vi "WS1050_Extract Data From Scope_Filtered Signal.vi"(0 "file path":path=path "S:/_Employee_Folders/Andy temp/SN01/444AB_04__SN01_C1_S1_UP_Switch_Time_data.csv", 1 "60% Amp":dbl=0.6, 2 "95% Amp":dbl=0.95, 9 "Set Point for AMP":i32=7000, 11 "error in (no error)":errorcluster, 12 "90% Amp":dbl=0.9) -> (3 "AMP(v)":dbl=1.1, 4 "Amp(mv)":string, 6 "T2(us)":string, 8 "T3(us)":string, 10 "T1(us)":string, 15 "error out":errorcluster)   [LabVIEW 2012]
uses:
  <vilib>/Utility/file.llb/Read From Spreadsheet File (string).vi
  <vilib>/Analysis/2dsp.llb/Real FFT.vi
  <vilib>/Analysis/NI_AALPro.lvlib
panel:
  in  "Tab Control":enum32{"Control", "ST", "FFT"}(tab)
  in  "Enter Time(s)":dbl=0.0001
  in  "Full/Half":i32=2
  out "Signal":cluster{dbl, dbl}[](graph)
  out "Filtered Signal":cluster{dbl, dbl}[](graph)
  out "CLK":cluster{dbl, dbl}[](graph)
  out "Signal FFT":cluster{dbl, dbl}[](graph)
  out "Filtered Signal FFT":cluster{dbl, dbl}[](graph)
  # "Total Time is 10E-4"
  # "Note\nSample time is 10E-8\nTotal time is 10E-4"
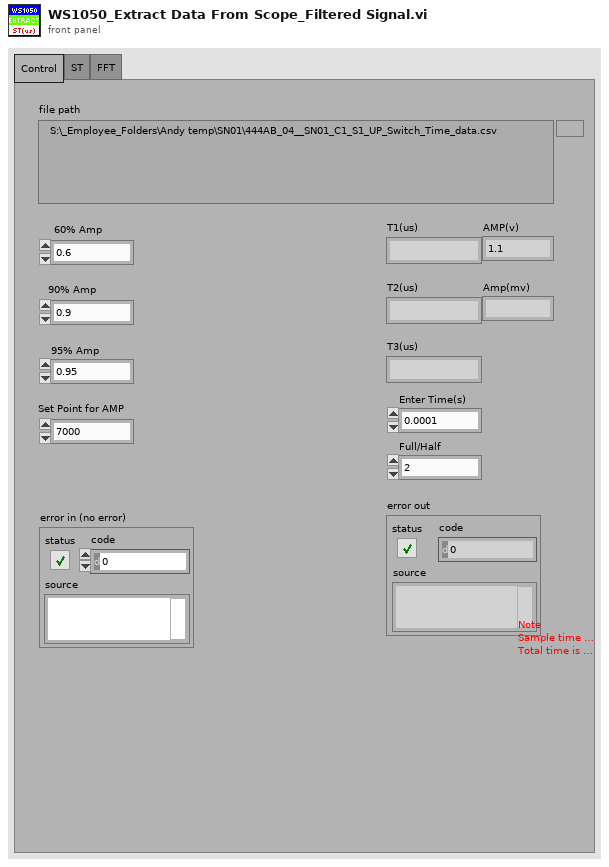
[diagram p1: front panel]
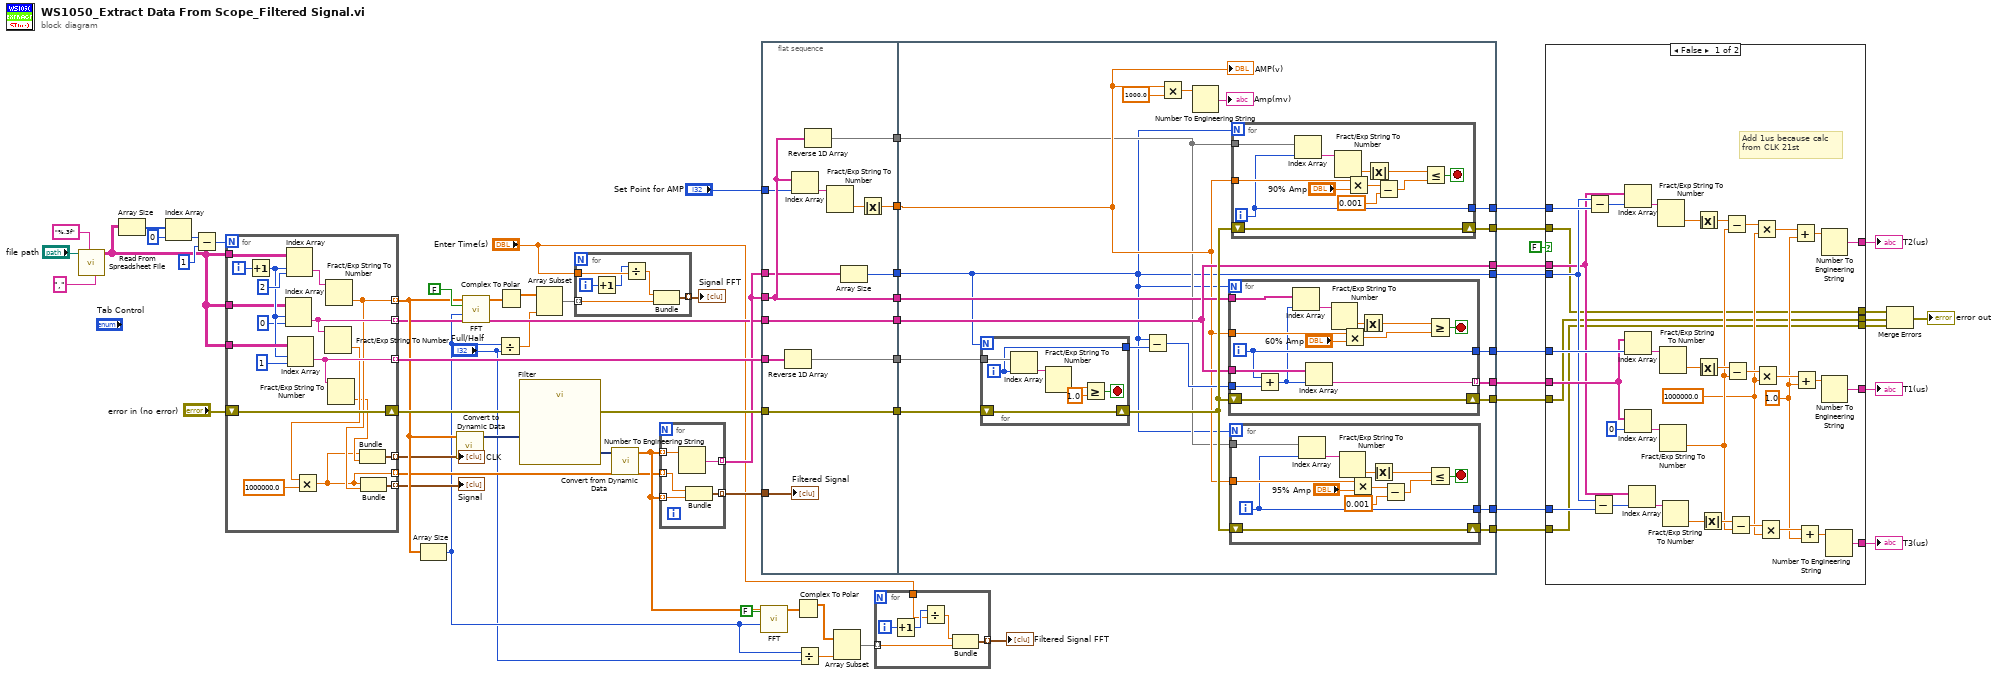
[diagram p0: block diagram]
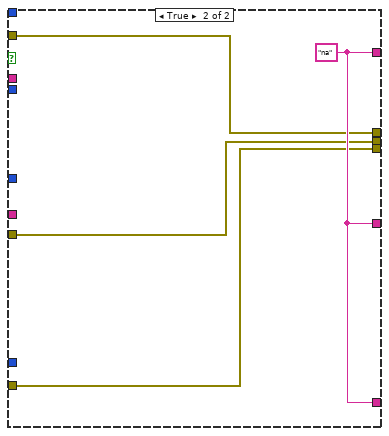
[diagram p2: hidden frame]
diagram:
  n1 = call-poly <vilib>:"Read From Spreadsheet File.vi"("delimiter (\\t)"="," ("delimiter (\\t)"), "format (%s)"="%.3f" ("format (%.3f)"), "file path (dialog if empty)"="file path") -> ("all rows"=w47:string[][])  [unwired: 4 in, 4 out]
  n2 = Array Size(array=w47) -> (size(s)=w60:i32[])
  n3 = Index Array(array=w60, index=0) -> (element=w58:i32)
  n4 = Subtract(x=w58, y=1) -> (x-y=w21:i32)
  n5 = for {
    N: w21 -> [_]
    tunnel: w47 -> [w82]
    tunnel: w47 -> [w79]
    tunnel: [w72] -> w55 mode=indexing
    tunnel: w47 -> [w76]
    tunnel: [w71] -> w18 mode=indexing
    shift-right: [w74] -> w30
    shift-left: "error in (no error)" -> [w74]
    tunnel: [w67] -> w19 mode=indexing
    tunnel: [w69] -> w16 mode=indexing
    tunnel: [w65] -> w14 mode=indexing
    tunnel: [w64] -> w12 mode=indexing
    i -> [w80]
    n6 = Increment(x=w80) -> (x+1=w77:i32)
    n7 = Index Array(array=w76, index (row)=w77, index (col)=0 ("disabled index (col)")) -> (element=w71:string)
    n8 = Index Array(array=w82, index (row)=w77, index (col)=2 ("disabled index (col)")) -> (element=w73:string)
    n9 = Index Array(array=w79, index (row)=w77, index (col)=1 ("disabled index (col)")) -> (element=w72:string)
    n10 = Fract/Exp String To Number(string=w71) -> (number=w68:dbl)  [unwired: 3 in, 1 out]
    n11 = Multiply(x=w68, y=1000000.0) -> (x*y=w65:dbl)
    n12 = Fract/Exp String To Number(string=w73) -> (number=w67:dbl)  [unwired: 3 in, 1 out]
    n13 = Fract/Exp String To Number(string=w72) -> (number=w66:dbl)  [unwired: 3 in, 1 out]
    n14 = Bundle(w65, w66) -> (w64:cluster{dbl, dbl})  [unwired: 1 in]
    n15 = Bundle(w65, w67) -> (w69:cluster{dbl, dbl})  [unwired: 1 in]
  }
  "Signal" <- w16
  "CLK" <- w12
  n16 = Array Size(array=w19) -> (size(s)=w4:i32)
  n17 = call "Convert to Dynamic Data"("Array"=w19) -> ("Dynamic Data Type"=w29:dynamicdata)  [unwired: 3 in]
  n18 = call-poly <vilib>:"FFT.vi"("FFT size"=w4, "shift?"=FALSE, "X"=w19) -> ("FFT {X}"=w24:cdb[])  [unwired: 7 in, 1 out]
  n19 = Divide(x=w4, y="Full/Half") -> (x/y=w3:dbl)
  n20 = Complex To Polar(r * e^(i*theta)=w24) -> (r=w6:dbl[])  [unwired: 1 out]
  n21 = call "Filter"("error in (no error)"=w30, "Signal"=w29) -> ("error out"=w28:errorcluster, "Filtered Signal"=w27:dynamicdata)  [unwired: 8 in]
  n22 = Array Subset(array=w6, length=w3) -> (w5:dbl[])  [unwired: 1 in]
  n23 = for {
    tunnel: w5 -> [w88] mode=indexing
    tunnel: [w87] -> w11 mode=indexing
    tunnel: "Enter Time(s)" -> [w84]
    i -> [w86]
    n24 = Increment(x=w86) -> (x+1=w83:i32)
    n25 = Divide(x=w83, y=w84) -> (x/y=w85:dbl)
    n26 = Bundle(w85, w88) -> (w87:cluster{dbl, dbl})  [unwired: 1 in]
  }
  "Signal FFT" <- w11
  n27 = call "Convert from Dynamic Data"("Dynamic Data Type"=w27) -> ("Array"=w15:dbl[])  [unwired: 3 in]
  n28 = for {
    tunnel: w15 -> [w93] mode=indexing
    tunnel: [w92] -> w26 mode=indexing
    tunnel: w15 -> [w91] mode=indexing
    tunnel: w14 -> [w90] mode=indexing
    tunnel: [w89] -> w13 mode=indexing
    n29 = Number To Engineering String(4:w93) -> (0:w92:string)  [unwired: 3 in]
    n30 = Bundle(w90, w91) -> (w89:cluster{dbl, dbl})  [unwired: 1 in]
  }
  n31 = call-poly <vilib>:"FFT.vi"("FFT size"=w4, "shift?"=FALSE, "X"=w15) -> ("FFT {X}"=w20:cdb[])  [unwired: 7 in, 1 out]
  n32 = flat-sequence {
    tunnel: w18 -> [w105]
    tunnel: w28 -> [w106]
    tunnel: w55 -> [w101]
    tunnel: [w106] -> w37
    tunnel: [w105] -> w36
    tunnel: w26 -> [w98]
    tunnel: [w102] -> w35
    tunnel: [w100] -> w34
    tunnel: [w99] -> w33
    tunnel: [w98] -> w32
    tunnel: [w97] -> w31
    tunnel: w26 -> [w96]
    tunnel: "Set Point for AMP" -> [w95]
    tunnel: w13 -> [w94]
    tunnel: [w126] -> w56
    tunnel: [w124] -> w52
    tunnel: [w123] -> w51
    tunnel: [w119] -> w49
    tunnel: [w118] -> w48
    tunnel: [w107] -> w43
    tunnel: [w113] -> w42
    tunnel: [w115] -> w46
    tunnel: [w114] -> w44
    tunnel: w37 -> [w125]
    tunnel: w36 -> [w113]
    tunnel: w35 -> [w110]
    tunnel: w34 -> [w109]
    tunnel: w33 -> [w108]
    tunnel: w32 -> [w111]
    tunnel: w31 -> [w107]
    frame #0 {
      n33 = Reverse 1D Array(array=w101) -> (reversed array=w100:string[])
      n34 = Index Array(array=w98, index=w95) -> (element=w103:string)
      n35 = Reverse 1D Array(array=w98) -> (reversed array=w99:string[])
      n36 = Fract/Exp String To Number(string=w103) -> (number=w104:dbl)  [unwired: 3 in, 1 out]
      n37 = Array Size(array=w96) -> (size(s)=w97:i32)
      n38 = Absolute Value(x=w104) -> (abs(x)=w102:dbl)
      "Filtered Signal" <- w94
    }
    frame #1 {
      n39 = for {
        N: w107 -> [_]
        tunnel: w109 -> [w171]
        tunnel: [w168] -> w117
        shift-right: [w166] -> w116
        shift-left: w125 -> [w166]
        i -> [w168]
        stop <- w169 stop-if-true
        n40 = Index Array(array=w171, index=w168) -> (element=w165:string)
        n41 = Fract/Exp String To Number(string=w165) -> (number=w167:dbl)  [unwired: 3 in, 1 out]
        n42 = Greater Or Equal?(x=w167, y=1.0) -> (x >= y?=w169:bool)
      }
      n43 = Subtract(x=w107, y=w117) -> (x-y=w112:i32)
      n44 = Multiply(x=w110, y=1000.0) -> (x*y=w121:dbl)
      n45 = Number To Engineering String(4:w121) -> (0:→"Amp(mv)":string)  [unwired: 3 in]
      n46 = for {
        N: w107 -> [_]
        tunnel: w111 -> [w164]
        tunnel: w110 -> [w162]
        tunnel: w113 -> [w161]
        tunnel: [w160] -> w118 mode=indexing
        tunnel: [w157] -> w126
        tunnel: w112 -> [w159]
        shift-right: [w154] -> w123
        shift-left: w116 -> [w154]
        i -> [w157]
        stop <- w163 stop-if-true
        n47 = Add(x=w157, y=w159) -> (x+y=w156:i32)
        n48 = Index Array(array=w164, index=w156) -> (element=w158:string)
        n49 = Index Array(array=w161, index=w156) -> (element=w160:string)
        n50 = Fract/Exp String To Number(string=w158) -> (number=w153:dbl)  [unwired: 3 in, 1 out]
        n51 = Multiply(x=w162, y="60% Amp") -> (x*y=w151:dbl)
        n52 = Absolute Value(x=w153) -> (abs(x)=w152:dbl)
        n53 = Greater Or Equal?(x=w152, y=w151) -> (x >= y?=w163:bool)
      }
      n54 = for {
        N: w107 -> [_]
        tunnel: w108 -> [w138]
        tunnel: w110 -> [w136]
        tunnel: [w132] -> w114
        shift-right: [w134] -> w115
        shift-left: w116 -> [w134]
        i -> [w132]
        stop <- w137 stop-if-true
        n55 = Index Array(array=w138, index=w132) -> (element=w131:string)
        n56 = Fract/Exp String To Number(string=w131) -> (number=w133:dbl)  [unwired: 3 in, 1 out]
        n57 = Multiply(x=w136, y="95% Amp") -> (x*y=w129:dbl)
        n58 = Absolute Value(x=w133) -> (abs(x)=w130:dbl)
        n59 = Subtract(x=w129, y=0.001) -> (x-y=w128:dbl)
        n60 = Less Or Equal?(x=w130, y=w128) -> (x <= y?=w137:bool)
      }
      n61 = for {
        N: w107 -> [_]
        tunnel: w108 -> [w150]
        tunnel: w110 -> [w148]
        tunnel: [w144] -> w119
        shift-right: [w146] -> w124
        shift-left: w116 -> [w146]
        i -> [w144]
        stop <- w149 stop-if-true
        n62 = Index Array(array=w150, index=w144) -> (element=w143:string)
        n63 = Fract/Exp String To Number(string=w143) -> (number=w145:dbl)  [unwired: 3 in, 1 out]
        n64 = Multiply(x=w148, y="90% Amp") -> (x*y=w141:dbl)
        n65 = Absolute Value(x=w145) -> (abs(x)=w142:dbl)
        n66 = Subtract(x=w141, y=0.001) -> (x-y=w140:dbl)
        n67 = Less Or Equal?(x=w142, y=w140) -> (x <= y?=w149:bool)
      }
      "AMP(v)" <- w110
    }
  }
  n68 = Complex To Polar(r * e^(i*theta)=w20) -> (r=w7:dbl[])  [unwired: 1 out]
  n69 = Divide(x=w4, y="Full/Half") -> (x/y=w2:dbl)
  n70 = Array Subset(array=w7, length=w2) -> (w8:dbl[])  [unwired: 1 in]
  n71 = for {
    tunnel: w8 -> [w177] mode=indexing
    tunnel: [w176] -> w9 mode=indexing
    tunnel: "Enter Time(s)" -> [w172]
    i -> [w175]
    n72 = Increment(x=w175) -> (x+1=w173:i32)
    n73 = Divide(x=w173, y=w172) -> (x/y=w174:dbl)
    n74 = Bundle(w174, w177) -> (w176:cluster{dbl, dbl})  [unwired: 1 in]
  }
  "Filtered Signal FFT" <- w9
  n75 = case shown="False" FALSE {
    tunnel: w56 -> [w211 _]
    tunnel: [w209 w218] -> w53
    tunnel: w52 -> [w180 w217]
    tunnel: w51 -> [w179 w216]
    tunnel: [w208 w218] -> w50
    tunnel: w49 -> [w197 _]
    tunnel: w48 -> [w196 _]
    tunnel: w46 -> [w178 w215]
    tunnel: [w187 w218] -> w45
    tunnel: w44 -> [w186 _]
    tunnel: w43 -> [w185 _]
    tunnel: w42 -> [w184 _]
    tunnel: [w180 w217] -> w41
    tunnel: [w179 w216] -> w40
    tunnel: [w178 w215] -> w39
    frame False {
      w181 = 1.0 ("y")
      w182 = 1000000.0 ("y")
      # "Add 1us because calc \nfrom CLK 21st"
      n76 = Subtract(x=w185, y=w197) -> (x-y=w195:i32)
      n77 = Subtract(x=w185, y=w186) -> (x-y=w194:i32)
      n78 = Index Array(array=w184, index=w195) -> (element=w206:string)
      n79 = Index Array(array=w196, index=w211) -> (element=w214:string)
      n80 = Index Array(array=w196, index=0) -> (element=w212:string)
      n81 = Index Array(array=w184, index=w194) -> (element=w189:string)
      n82 = Fract/Exp String To Number(string=w206) -> (number=w200:dbl)  [unwired: 3 in, 1 out]
      n83 = Fract/Exp String To Number(string=w214) -> (number=w198:dbl)  [unwired: 3 in, 1 out]
      n84 = Fract/Exp String To Number(string=w212) -> (number=w183:dbl)  [unwired: 3 in, 1 out]
      n85 = Fract/Exp String To Number(string=w189) -> (number=w193:dbl)  [unwired: 3 in, 1 out]
      n86 = Absolute Value(x=w200) -> (abs(x)=w201:dbl)
      n87 = Absolute Value(x=w198) -> (abs(x)=w199:dbl)
      n88 = Absolute Value(x=w193) -> (abs(x)=w192:dbl)
      n89 = Subtract(x=w201, y=w183) -> (x-y=w207:dbl)
      n90 = Subtract(x=w199, y=w183) -> (x-y=w210:dbl)
      n91 = Subtract(x=w192, y=w183) -> (x-y=w188:dbl)
      n92 = Multiply(x=w207, y=w182) -> (x*y=w202:dbl)
      n93 = Multiply(x=w210, y=w182) -> (x*y=w204:dbl)
      n94 = Multiply(x=w188, y=w182) -> (x*y=w191:dbl)
      n95 = Add(x=w202, y=w181) -> (x+y=w203:dbl)
      n96 = Add(x=w204, y=w181) -> (x+y=w205:dbl)
      n97 = Add(x=w191, y=w181) -> (x+y=w190:dbl)
      n98 = Number To Engineering String(4:w203) -> (0:w208:string)  [unwired: 3 in]
      n99 = Number To Engineering String(4:w205) -> (0:w209:string)  [unwired: 3 in]
      n100 = Number To Engineering String(4:w190) -> (0:w187:string)  [unwired: 3 in]
    }
    frame True {
      w218 = "na"
    }
  }
  "T1(us)" <- w53
  "T2(us)" <- w50
  "T3(us)" <- w45
  n101 = Merge Errors(w41, w40, w39) -> (→"error out":errorcluster)
